vi "CONEX-ALL Set Controller's address v2.vi"(9 "Controller's address":i32, 11 "Connection Cluster in":T1) -> (3 "Connection Cluster out":T1)   [LabVIEW 2010]
doc: "SA - Set controller's RS-485 address\n\nNOTE: For CONEX over USB the RS-485 Address will always be 1, this command will not change the address. Each USB bus (cable) only talks to the attached device, not to any other device. Therefore, having the option of changing the address is not needed.\n\nInput: New address for controller\n\nOutput: New address will be set in Connection cluster."
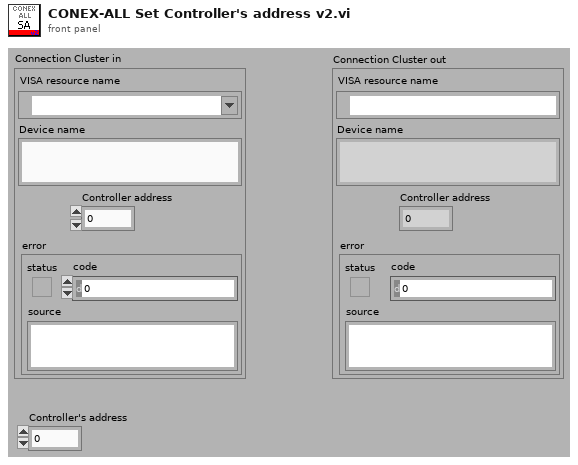
[diagram p1: front panel]
types:
  T1 = cluster{"VISA resource name":refnum<visa-resource-name>, "Device name":string, "Controller address":i32, "error":errorcluster}
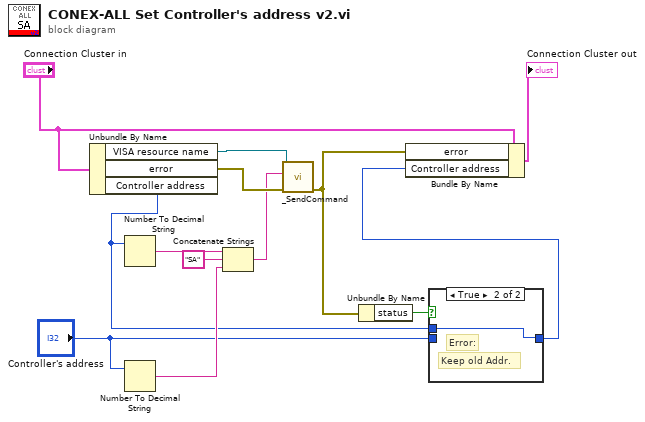
[diagram p0: block diagram]
diagram:
  n1 = Unbundle By Name("Connection Cluster in") -> ("VISA resource name"=w8:refnum<visa-resource-name>, "error"=w7:errorcluster, "Controller address"=w1:i32)
  n2 = Number To Decimal String(number=w1) -> (decimal integer string=w13:string)  [unwired: 1 out]
  n3 = Number To Decimal String(number="Controller's address") -> (decimal integer string=w11:string)  [unwired: 1 in]
  n4 = Concatenate Strings(w13, "SA" ("strCommand"), w11) -> (w4:string)
  n5 = call <userlib>:"_SendCommand.vi"("error in"=w7, "Command"=w4, "Instrument Channel"=w8) -> ("error out"=w3:errorcluster)  [unwired: 7 in, 1 out]
  n6 = Unbundle By Name(w3) -> ("status"=w10:bool)
  n7 = case shown="True" w10 {
    tunnel: "Controller's address" -> [w14 _]
    tunnel: [w14 w15] -> w2
    tunnel: w1 -> [_ w15]
    frame False {
    }
    frame True {
      # "Error:"
      # "Keep old Addr."
    }
  }
  n8 = Bundle By Name(cluster="Connection Cluster in", "error"=w3, "Controller address"=w2) -> (→"Connection Cluster out":T1)
